vi "Create.vi"(8 "error in":errorcluster, 10 "Main VI Path":path) -> (0 "error out":errorcluster, 3 "Master Reference":T1)   [LabVIEW 2021, in "RT Interpreter.lvlib" / "VI Reference Management.lvlib"]
doc: "Create the master VI reference for the cloneable Main VI.\n_____\nBased on DQMH Dev Tools: Project Template 7.1.2.1547."
uses:
  VI Reference Management.lvlib
  Main VI Type--strict_vi_ref.ctl
  <vilib>/Delacor/Delacor QMH/Libraries/Cloneable Module Admin_class/Delacor_lib_QMH_Cloneable Module Admin.lvclass
  Action--enum.ctl
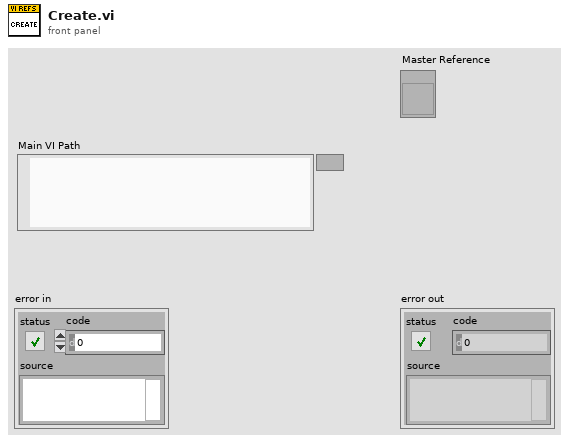
[diagram p1: front panel]
types:
  T1 = typedef "RT Interpreter.lvlib/VI Reference Management.lvlib/Main VI Type--strict_vi_ref.ctl" = refnum<vi>
  T2 = typedef "RT Interpreter.lvlib/VI Reference Management.lvlib/Action--enum.ctl" = enum16{"Get", "Create", "Close"}
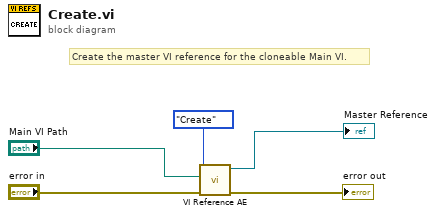
[diagram p0: block diagram]
diagram:
  # "Create the master VI reference for the cloneable Main VI."
  n1 = call "VI Reference AE.vi"("error in"="error in", "Main VI Path"="Main VI Path", "Action"=Action--enum."Create") -> ("error out"=→"error out":errorcluster, "Master Reference"=→"Master Reference":T1)  [unwired: 6 in]
